vi "Send Centrialize Error Handling.vi"(7 "Message Priority (Normal)":T2=enum."Normal", 8 "error in (no error)":errorcluster, 9 "Error":errorcluster, 10 "Error Level":T1, 11 "Message Enqueuer":refnum<class "Message Enqueuer.lvclass">) -> (0 "error out":errorcluster, 3 "Message Enqueuer out":refnum<class "Message Enqueuer.lvclass">)   [LabVIEW 2019, in "Car Wash Controller Actor.lvlib" / "Centrialize Error Handling Msg.lvclass"]
doc: "This VI sends the message to an actor."
uses:
  Centrialize Error Handling Msg.lvclass
  <vilib>/ActorFramework/Message Enqueuer/Message Enqueuer.lvclass
  <vilib>/ActorFramework/Message Enqueuer/Message Priority.ctl
  Car Wash Controller Actor/Error Levels.ctl
  C:/Program Files (x86)/National Instruments/LabVIEW 2019/vi.lib/ActorFramework/Message/Message.lvclass
  Centrialize Error Handling Msg.lvclass/Centrialize Error Handling Msg.ctl
  <vilib>/ActorFramework/Message Enqueuer/Message Enqueuer.lvclass/Message Enqueuer.ctl
  <vilib>/ActorFramework/Message Priority Queue/Priority Enqueue.vi
  Car Wash Controller Actor/Car Wash Controller Actor.lvclass
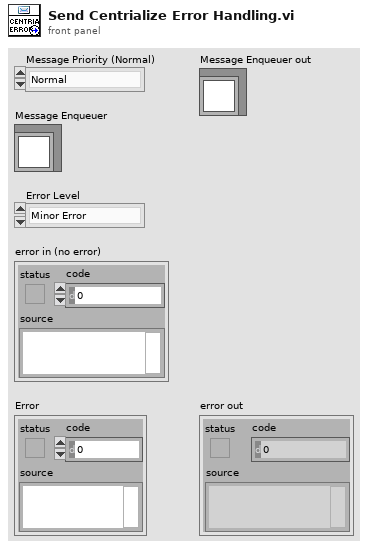
[diagram p1: front panel]
types:
  T1 = typedef "Car Wash Controller Actor.lvlib/Car Wash Controller Actor.lvclass/Error Levels.ctl" = enum16{"Minor Error", "Wash Cycle Error", "System Error"}
  T2 = typedef "Actor Framework.lvlib/Message Enqueuer.lvclass/Message Priority.ctl" = enum16{"Low", "Normal", "High"}
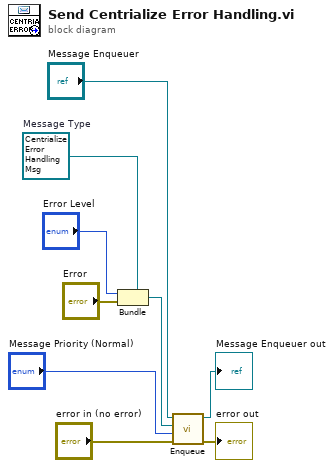
[diagram p0: block diagram]
diagram:
  w6 = refnum<class "Centrialize Error Handling Msg.lvclass"> refnum  # Message Type
  n1 = Bundle(cluster=w6, "Error Level", "Error") -> (w5:refnum<class "Centrialize Error Handling Msg.lvclass">)
  n2 = call <vilib>:"Enqueue.vi"("error in (no error)"="error in (no error)", "Message Priority (Normal)"="Message Priority (Normal)", "Message"=w5, "Message Enqueuer in"="Message Enqueuer") -> ("error out"=→"error out":errorcluster, "Message Enqueuer out"=→"Message Enqueuer out":refnum<class "Message Enqueuer.lvclass">)  [unwired: 6 in]
